vi "Observe Data.vi"(6 "Time Stamp":timestamp, 8 "error in (no error)":errorcluster, 9 "Value":variant, 10 "Datum Name":string, 11 "ModelSubscribesToDoubleFloatX in":refnum<class "ModelSubscribesToDoubleFloatX.lvclass">) -> (0 "error out":errorcluster, 3 "ModelSubscribesToDoubleFloatX out":refnum<class "ModelSubscribesToDoubleFloatX.lvclass">)   [LabVIEW 2017, in "ModelSubscribesToDoubleFloatX.lvclass"]
doc: "<License>\nCopyright © 2017 Composed Systems, LLC | All rights reserved\nwww.composed.io\n\nAuthor: Ethan Stern <ethan.stern@composed.io>\n\nThis software is provided \"AS IS\" WITHOUT WARRANTIES, either express or implied, AND IS FOR EDUCATIONAL PURPOSES ONLY.\n</License>"
uses:
  ModelSubscribesToDoubleFloatX.lvclass
  ModelSubscribesToDoubleFloatX.lvclass/ModelSubscribesToDoubleFloatX.ctl
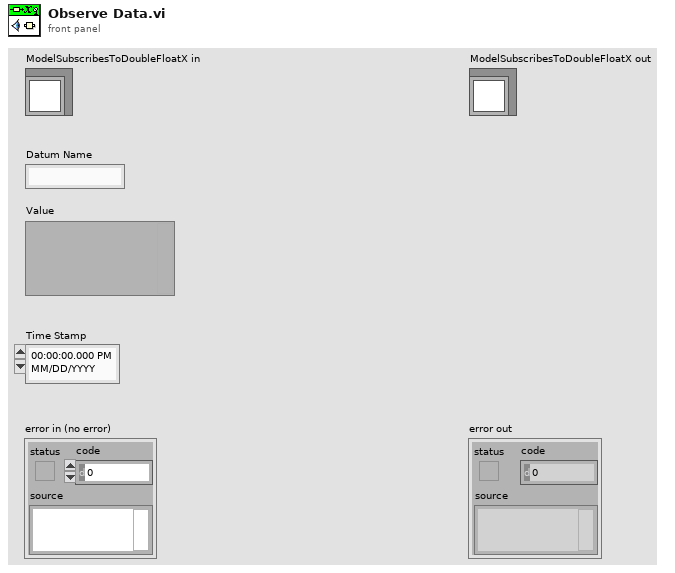
[diagram p1: front panel]
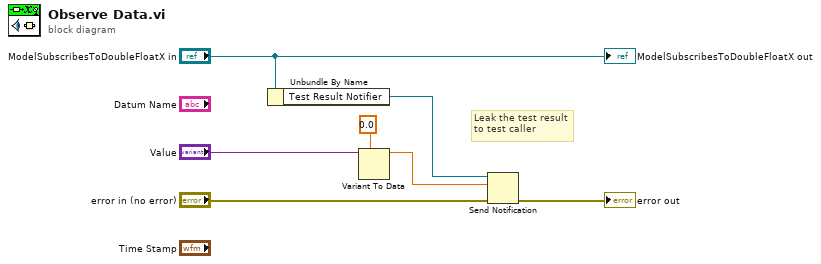
[diagram p0: block diagram]
diagram:
  # "Leak the test result\nto test caller"
  n1 = Unbundle By Name("ModelSubscribesToDoubleFloatX in") -> ("Test Result Notifier"=w4:refnum<notifier>)
  n2 = Variant To Data(type=0.0, Variant="Value") -> (data=w2:dbl)  [unwired: 1 in, 1 out]
  n3 = Send Notification(notification=w2, notifier=w4, error in (no error)="error in (no error)") -> (error out=→"error out":errorcluster)  [unwired: 1 out]
  "ModelSubscribesToDoubleFloatX out" <- "ModelSubscribesToDoubleFloatX in"
